vi "WriteEvtConfig.vi"(8 "error in (no error)":errorcluster, 10 "Event Configuration":T1={"UTC Time 0"=timestamp(0 s since 1904-01-01), "Nominal Frequency"=60, "Reporting Rate"=60, "Fsamp"=960, "PosSeq"=FALSE} {"Reporting Rate" items=["10 FPS"=10, "12 FPS"=12, "15 FPS"=15, "20 FPS"=20, "25 FPS"=25, "30 FPS"=30, "50 FPS"=50, "60 FPS"=60]; "Nominal Frequency" items=["50 Hz"=50, "60 Hz"=60]}, 11 "LSEPlugin in":refnum<class "LSEPlugin.lvclass">) -> (0 "error out":errorcluster, 3 "LSEPlugin out":refnum<class "LSEPlugin.lvclass">)   [LabVIEW 2014, in "AppPlugins.lvlib" / "LSEPlugin.lvclass"]
uses:
  LSEPlugin.lvclass
  Framework/FrontPanel/TypeDefs/clEventConfig.ctl
  LSEPlugin.lvclass/LSEPlugin.ctl
  Accessors/Read LSEConfig.vi
  Framework/Framework.lvlib
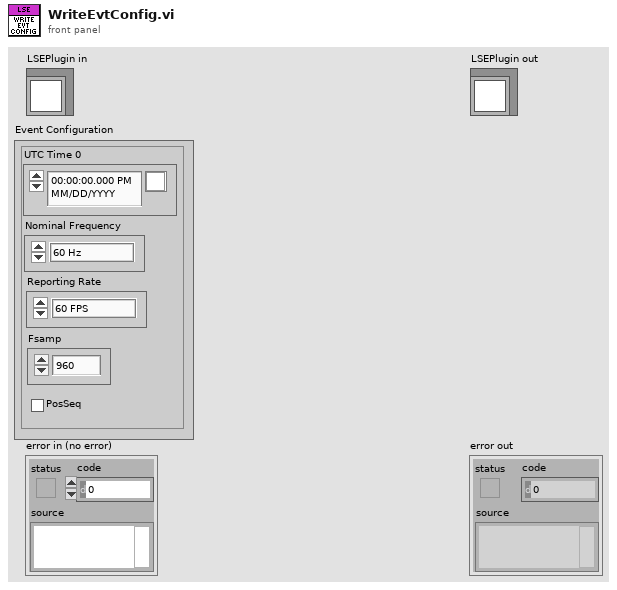
[diagram p1: front panel]
types:
  T1 = typedef "Framework.lvlib/clEventConfig.ctl" = cluster{"UTC Time 0":timestamp, "Nominal Frequency":u16, "Reporting Rate":u16, "Fsamp":u32, "PosSeq":bool}
  T2 = typedef "AppPlugins.lvlib/LSEPlugin.lvclass/LSEConfig.ctl" = cluster{"NoiseVariance":dbl, "IEEESystem":u32, "PMULocations":u32[], "Vindex":i32, "Iindex":i32, "DynamicRef":string}
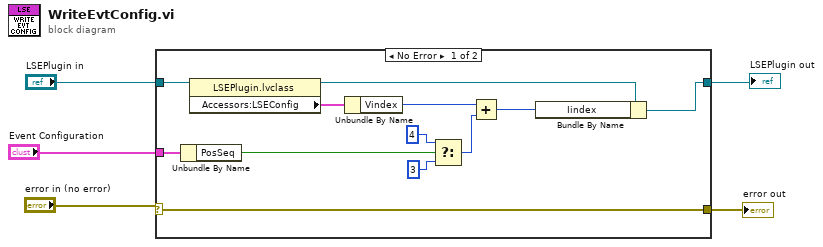
[diagram p0: block diagram]
diagram:
  n1 = case shown="No Error" "error in (no error)" {
    selector: "error in (no error)" -> [w7 w18]
    tunnel: "LSEPlugin in" -> [w16 w19]
    tunnel: [w8 w19] -> w4
    tunnel: [w7 w18] -> w3
    tunnel: "Event Configuration" -> [w17 _]
    frame No Error {
      n2 = Unbundle By Name(w17) -> ("PosSeq"=w6:bool)
      n3 = property class="LSEPlugin.lvclass"(reference=w16) -> (reference out=w10:refnum<class "LSEPlugin.lvclass">, "Accessors:LSEConfig"=w15:T2)  [unwired: 1 in, 1 out]
      n4 = Unbundle By Name(w15) -> ("Vindex"=w11:i32)
      n5 = Select(t=4, s=w6, f=3) -> (s? t:f=w12:i32)
      n6 = Add(x=w11, y=w12) -> (x+y=w9:i32)
      n7 = Bundle By Name(cluster=w10, "Iindex"=w9) -> (w8:refnum<class "LSEPlugin.lvclass">)
    }
    frame Error {
    }
  }
  "error out" <- w3
  "LSEPlugin out" <- w4
